vi "Resolve UI Dependencies.vi"(8 "error in":errorcluster, 11 "Template Project Path":path) -> (0 "error out":errorcluster)   [LabVIEW 2021, in "Plugin Generator.lvlib"]
uses:
  Plugin Generator.lvlib
  <vilib>/Utility/traverseref.llb/TRef TravTarget.ctl
  <vilib>/Utility/traverseref.llb/VI Scripting - Traverse.lvlib
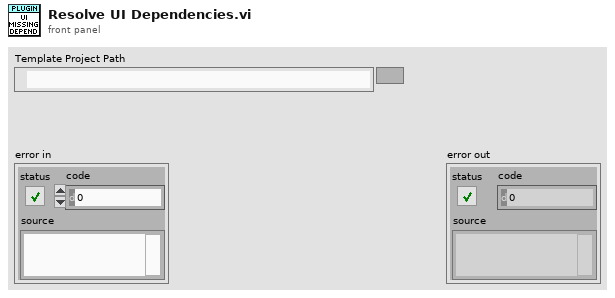
[diagram p1: front panel]
types:
  T1 = typedef "TRef TravTarget.ctl" = enum16{"FP", "BD", "Other"}
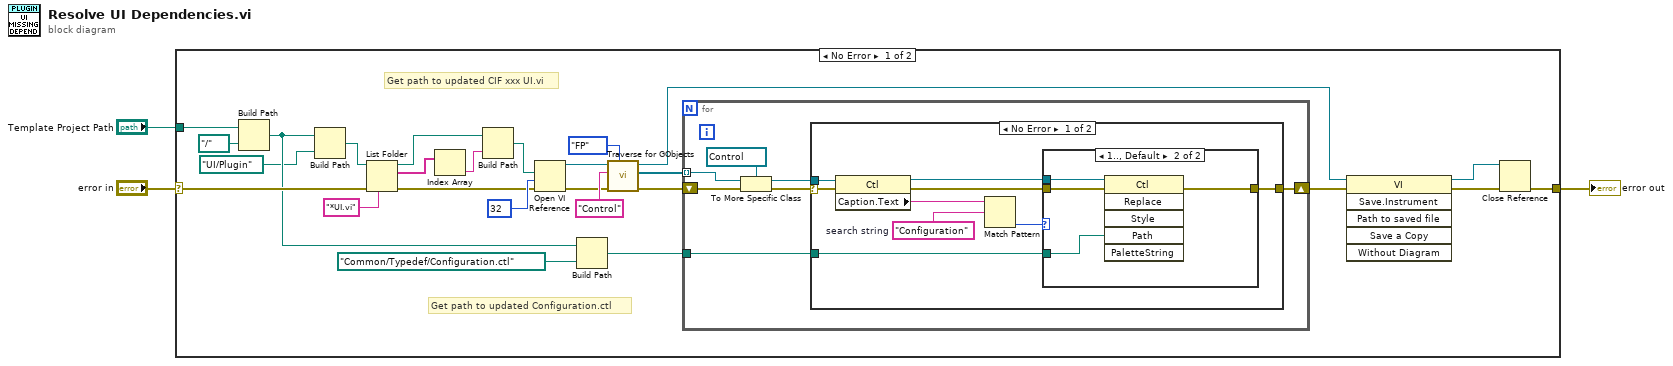
[diagram p0: block diagram]
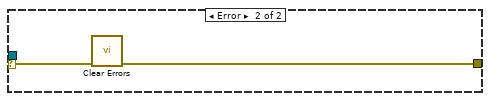
[diagram p3: hidden frame]
diagram:
  n1 = case shown="No Error" "error in" {
    selector: "error in" -> [w27 w53]
    tunnel: [w13 w53] -> w3
    tunnel: "Template Project Path" -> [w29 _]
    frame No Error {
      # "Get path to updated Configuration.ctl"
      # "Get path to updated CIF xxx UI.vi"
      n2 = Build Path(base path=w29, name or relative path=path "../..") -> (appended path=w6:path)
      n3 = Build Path(base path=w6, name or relative path=path "UI/Plugin") -> (appended path=w4:path)
      n4 = List Folder(path=w4, pattern="*UI.vi" ("Class Name"), error in=w27) -> (path out=w26:path, filenames=w25:string[], error out=w10:errorcluster)  [unwired: 1 in, 1 out]
      n5 = Index Array(array=w25) -> (element=w24:string)  [unwired: 1 in]
      n6 = Build Path(base path=w26, name or relative path=w24) -> (appended path=w9:path)
      n7 = Open VI Reference(vi path=w9, options=32, error in (no error)=w10) -> (vi reference=w12:refnum<vi>, error out=w11:errorcluster)  [unwired: 3 in]
      n8 = Build Path(base path=w6, name or relative path=path "Common/Typedef/Configuration.ctl") -> (appended path=w17:path)
      n9 = call <vilib>:"Traverse for GObjects.vi"("Traverse Target"=TRef_TravTarget."FP", "error in (no error)"=w11, "Class Name"="Control", "VI Refnum"=w12) -> ("error out"=w18:errorcluster, "References"=w21:refnum<vi>[], "dup VI Refnum"=w8:refnum<vi>)  [unwired: 4 in, 1 out]
      n10 = for {
        tunnel: w21 -> [w36] mode=indexing
        shift-right: [w34] -> w16
        shift-left: w18 -> [w32]
        tunnel: w17 -> [w31]
        n11 = To More Specific Class(target class=refnum<vi> refnum ("x"), reference=w36, error in=w32) -> (specific class reference=w33:refnum<vi>, error out=w30:errorcluster)
        n12 = case shown="No Error" w30 {
          selector: w30 -> [w37 w52]
          tunnel: [w43 w51] -> w34
          tunnel: w33 -> [w42 _]
          tunnel: w31 -> [w40 _]
          frame No Error {
            w39 = "Configuration"  # search string
            n13 = property class="Ctl"(reference=w42, error in=w37) -> (reference out=w44:refnum<vi>, error out=w45:errorcluster, "Caption.Text"=w41:string)
            n14 = Match Pattern(string=w41, regular expression=w39) -> (offset past match=w38:i32)  [unwired: 1 in, 3 out]
            n15 = case shown="1.., Default" w38 {
              tunnel: w45 -> [w46 w48]
              tunnel: w44 -> [_ w47]
              tunnel: [w46 w50] -> w43
              tunnel: w40 -> [_ w49]
              frame -1 {
              }
              frame 1.., Default {
                n16 = invoke class="Ctl" method="Replace"(reference=w47, error in=w48, "Path"=w49) -> (error out=w50:errorcluster)  [unwired: 3 in, 5 out]
              }
            }
          }
          frame Error {
            n17 = call <vilib>:"Clear Errors.vi"("error in (no error)"=w52) -> ("error out"=w51:errorcluster)  [unwired: 5 in, 1 out]
          }
        }
      }
      n18 = invoke class="VI" method="Save.Instrument"(reference=w8, error in=w16) -> (reference out=w14:refnum<vi>, error out=w15:errorcluster)  [unwired: 4 in, 4 out]
      n19 = Close Reference(reference=w14, error in (no error)=w15) -> (error out=w13:errorcluster)
    }
    frame Error {
    }
  }
  "error out" <- w3
